vi "Close Ref.vi"(8 "Error In":errorcluster, 11 "DVR Ref":refnum<data-value>) -> (0 "Error Out":errorcluster)   [LabVIEW 2019, in "Arithemetic Operation.lvclass"]
doc: "The method accepts the DVR of class data as the input and closes the VI reference that the class holds."
uses:
  Arithemetic Operation.lvclass
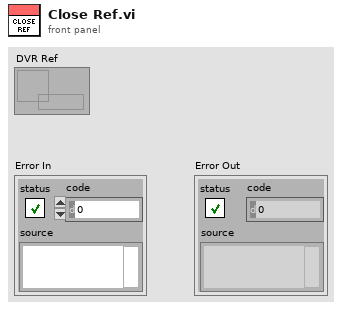
[diagram p1: front panel]
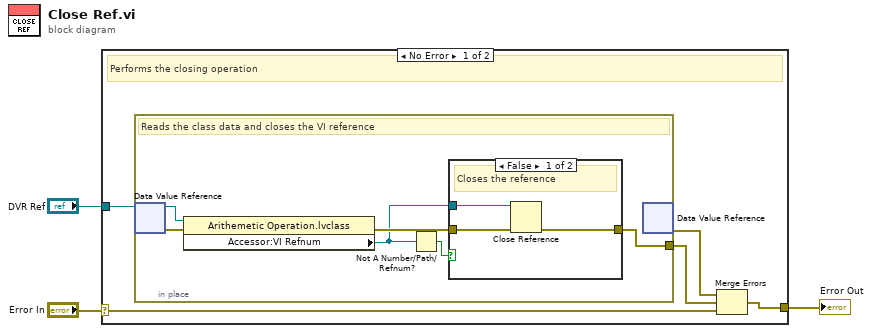
[diagram p0: block diagram]
diagram:
  n1 = case shown="No Error" "Error In" {
    selector: "Error In" -> [w5 w19]
    tunnel: "DVR Ref" -> [w8 _]
    tunnel: [w4 w19] -> w1
    frame No Error {
      # "Performs the closing operation"
      n2 = in-place {
        in-place-border: [w9] -> w7
        # "Reads the class data and closes the VI reference"
        n3 = in-place-dvr #1(w8) -> (w11:refnum<class "Arithemetic Operation.lvclass">, w10:errorcluster)
        n4 = property class="Arithemetic Operation.lvclass"(reference=w11, error in=w10) -> (error out=w14:errorcluster, "Accessor:VI Refnum"=w12:refnum<vi>)  [unwired: 1 out]
        n5 = Not A Number/Path/Refnum?(number/path/refnum=w12) -> (NaN/Path/Refnum?=w13:bool)
        n6 = case shown="False" w13 {
          tunnel: w14 -> [w17 w18]
          tunnel: [w16 w18] -> w9
          tunnel: w12 -> [w15 _]
          frame False {
            # "Closes the reference"
            n7 = Close Reference(reference=w15, error in (no error)=w17) -> (error out=w16:errorcluster)
          }
          frame True {
          }
        }
        n8 = in-place-dvr #1() -> (w6:errorcluster)  [unwired: 1 in, 1 out]
      }
      n9 = Merge Errors(w6, w7, w5) -> (w4:errorcluster)
    }
    frame Error {
    }
  }
  "Error Out" <- w1
